vi "inheritance.vi"   [LabVIEW 2017]
uses:
  Classes/FileMerge/FileMerge.lvclass
  Classes/Datalog/DataLog.lvclass
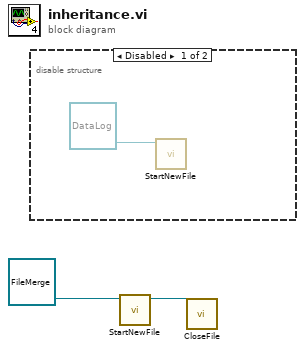
[diagram p0: block diagram]
diagram:
  n1 = disable-structure shown="Disabled" {
    frame Disabled {
      n2 = call-dynamic "StartNewFile.vi"("DataLog in"=refnum<class "DataLog.lvclass"> refnum) -> ()  [unwired: 9 in, 2 out]
    }
    frame Enabled {
    }
  }
  n3 = call-dynamic "StartNewFile.vi"("FileMerge in"=refnum<class "FileMerge.lvclass"> refnum ("FileMerge.lvclass")) -> ("FileMerge out"=w1:refnum<class "FileMerge.lvclass">)  [unwired: 9 in, 1 out]
  n4 = call-dynamic "CloseFile.vi"("FileMerge in"=w1) -> ()  [unwired: 9 in, 2 out]
